vi "Word_Font_Wizard.vi"(3 "error in (no error)":errorcluster, 4 "font in":T1={"font name"="", "font size"=0.0, "bold"=0, "italic"=0, "underline"=0, "strike through"=0, "font color"=16777216} caption="font" {"font size" format="%0.2f"; "strike through" items=["Unchanged", "Yes", "No"]; "underline" items=["Unchanged", "Yes", "No"]; "italic" items=["Unchanged", "Yes", "No"]; "bold" items=["Unchanged", "Yes", "No"]}, 5 "Word._Application":refnum<k7>) -> (0 "error out":errorcluster, 1 "font out":T1={"font name"="", "font size"=0.0, "bold"=0, "italic"=0, "underline"=0, "strike through"=0, "font color"=16777216} caption="font" {"font size" format="%0.2f"; "strike through" items=["Unchanged", "Yes", "No"]; "underline" items=["Unchanged", "Yes", "No"]; "italic" items=["Unchanged", "Yes", "No"]; "bold" items=["Unchanged", "Yes", "No"]})   [LabVIEW 2020, in "NI_ReportGenerationToolkit.lvlib"]
uses:
  <vilib>/addons/_office/NI_ReportGenerationToolkit.lvlib
  <vilib>/addons/_office/_exclsub.llb/font.ctl
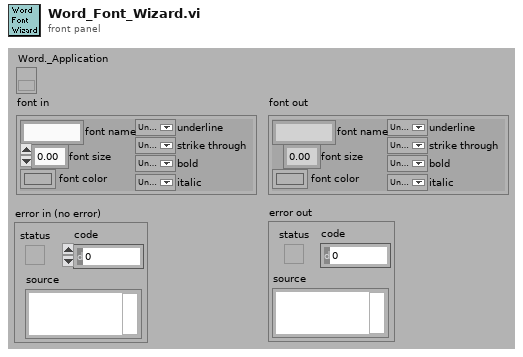
[diagram p1: front panel]
types:
  T1 = typedef "NI_ReportGenerationToolkit.lvlib/font.ctl" = cluster{"font name":string, "font size":dbl, "bold":u16, "italic":u16, "underline":u16, "strike through":u16, "font color":u32}
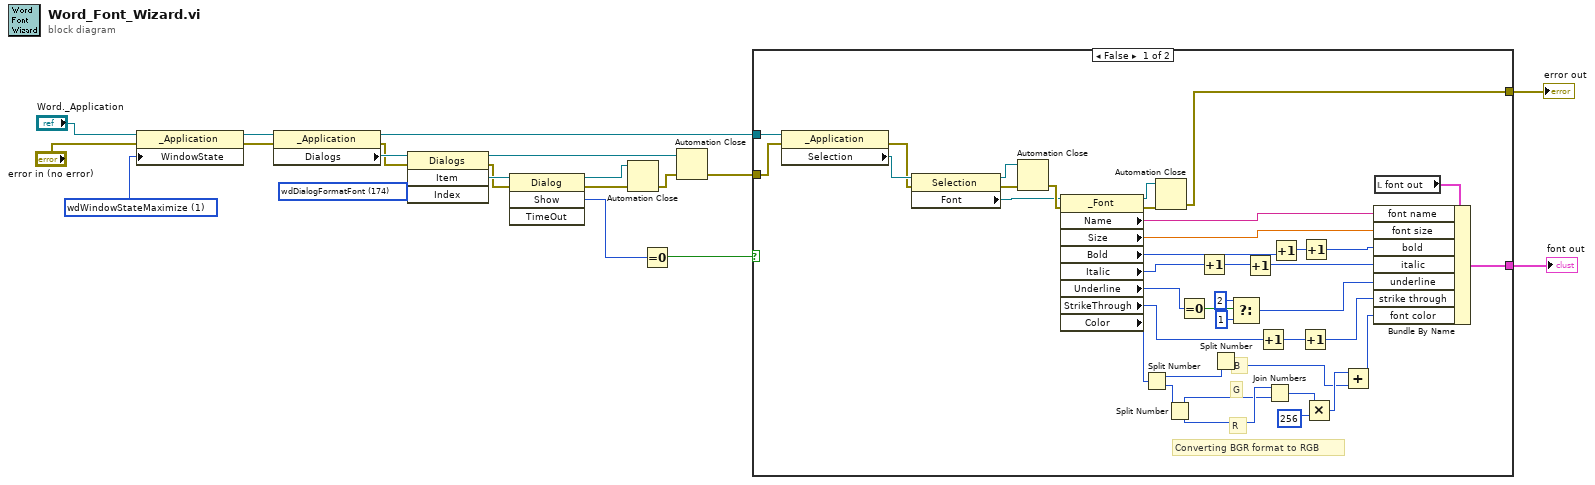
[diagram p0: block diagram]
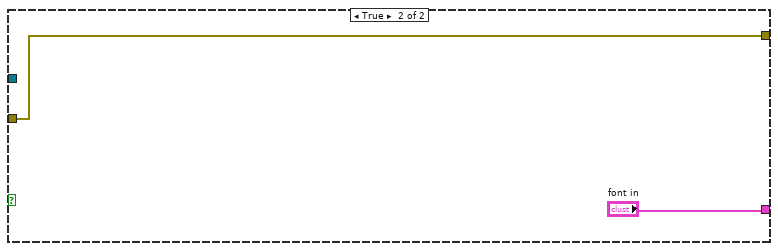
[diagram p2: hidden frame]
diagram:
  w6 = 1 items=["wdWindowStateNormal", "wdWindowStateMaximize", "wdWindowStateMinimize"] ("WindowState")
  w18 = 174 items=["wdDialogHelpAbout"=9, "wdDialogHelpWordPerfectHelp"=10, "wdDialogDocumentStatistics"=78, "wdDialogFileNew"=79, "wdDialogFileOpen"=80, "wdDialogMailMergeOpenDataSource"=81, "wdDialogMailMergeOpenHeaderSource"=82, "wdDialogFileSaveAs"=84, "wdDialogFileSummaryInfo"=86, "wdDialogToolsTemplates"=87, "wdDialogFilePrint"=88, "wdDialogFilePrintSetup"=97, "wdDialogFileFind"=99, "wdDialogFormatAddrFonts"=103, "wdDialogEditPasteSpecial"=111, "wdDialogEditFind"=112, "wdDialogEditReplace"=117, "wdDialogEditStyle"=120, "wdDialogEditLinks"=124, "wdDialogEditObject"=125, "wdDialogTableToText"=128, "wdDialogTextToTable"=127, "wdDialogTableInsertTable"=129, "wdDialogTableInsertCells"=130, "wdDialogTableInsertRow"=131, "wdDialogTableDeleteCells"=133, "wdDialogTableSplitCells"=137, "wdDialogTableRowHeight"=142, "wdDialogTableColumnWidth"=143, "wdDialogToolsCustomize"=152, "wdDialogInsertBreak"=159, "wdDialogInsertSymbol"=162, "wdDialogInsertPicture"=163, "wdDialogInsertFile"=164, "wdDialogInsertDateTime"=165, "wdDialogInsertField"=166, "wdDialogInsertMergeField"=167, "wdDialogInsertBookmark"=168, "wdDialogMarkIndexEntry"=169, "wdDialogInsertIndex"=170, "wdDialogInsertTableOfContents"=171, "wdDialogInsertObject"=172, "wdDialogToolsCreateEnvelope"=173, "wdDialogFormatFont"=174, "wdDialogFormatParagraph"=175, "wdDialogFormatSectionLayout"=176, "wdDialogFormatColumns"=177, "wdDialogFileDocumentLayout, wdDialogFilePageSetup"=178, "wdDialogFormatTabs"=179, "wdDialogFormatStyle"=180, "wdDialogFormatDefineStyleFont"=181, "wdDialogFormatDefineStylePara"=182, "wdDialogFormatDefineStyleTabs"=183, "wdDialogFormatDefineStyleFrame"=184, "wdDialogFormatDefineStyleBorders"=185, "wdDialogFormatDefineStyleLang"=186, "wdDialogFormatPicture"=187, "wdDialogToolsLanguage"=188, "wdDialogFormatBordersAndShading"=189, "wdDialogFormatFrame"=190, "wdDialogToolsThesaurus"=194, "wdDialogToolsHyphenation"=195, "wdDialogToolsBulletsNumbers"=196, "wdDialogToolsHighlightChanges, wdDialogToolsRevisions"=197, "wdDialogToolsCompareDocuments"=198, "wdDialogTableSort"=199, "wdDialogToolsOptionsGeneral"=203, "wdDialogToolsOptionsView"=204, "wdDialogToolsAdvancedSettings"=206, "wdDialogToolsOptionsPrint"=208, "wdDialogToolsOptionsSave"=209, "wdDialogToolsOptionsSpellingAndGrammar"=211, "wdDialogToolsOptionsUserInfo"=213, "wdDialogToolsMacroRecord"=214, "wdDialogToolsMacro"=215, "wdDialogWindowActivate"=220, "wdDialogFormatRetAddrFonts"=221, "wdDialogOrganizer"=222, "wdDialogToolsOptionsEdit"=224, "wdDialogToolsOptionsFileLocations"=225, "wdDialogToolsWordCount"=228, "wdDialogControlRun"=235, "wdDialogInsertPageNumbers"=294, "wdDialogFormatPageNumber"=298, "wdDialogCopyFile"=300, "wdDialogFormatChangeCase"=322, "wdDialogUpdateTOC"=331, "wdDialogInsertDatabase"=341, "wdDialogTableFormula"=348, "wdDialogFormFieldOptions"=353, "wdDialogInsertCaption"=357, "wdDialogInsertCaptionNumbering"=358, "wdDialogInsertAutoCaption"=359, "wdDialogFormFieldHelp"=361, "wdDialogInsertCrossReference"=367, "wdDialogInsertFootnote"=370, "wdDialogNoteOptions"=373, "wdDialogToolsAutoCorrect"=378, "wdDialogToolsOptionsTrackChanges"=386, "wdDialogConvertObject"=392, "wdDialogInsertAddCaption"=402, "wdDialogConnect"=420, "wdDialogToolsCustomizeKeyboard"=432, "wdDialogToolsCustomizeMenus"=433, "wdDialogToolsMergeDocuments"=435, "wdDialogMarkTableOfContentsEntry"=442, "wdDialogFileMacPageSetupGX"=444, "wdDialogFilePrintOneCopy"=445, "wdDialogEditFrame"=458, "wdDialogMarkCitation"=463, "wdDialogTableOfContentsOptions"=470, "wdDialogInsertTableOfAuthorities"=471, "wdDialogInsertTableOfFigures"=472, "wdDialogInsertIndexAndTables"=473, "wdDialogInsertFormField"=483, "wdDialogFormatDropCap"=488, "wdDialogToolsCreateLabels"=489, "wdDialogToolsProtectDocument"=503, "wdDialogFormatStyleGallery"=505, "wdDialogToolsAcceptRejectChanges"=506, "wdDialogHelpWordPerfectHelpOptions"=511, "wdDialogToolsUnprotectDocument"=521, "wdDialogToolsOptionsCompatibility"=525, "wdDialogTableOfCaptionsOptions"=551, "wdDialogTableAutoFormat"=563, "wdDialogMailMergeFindRecord"=569, "wdDialogReviewAfmtRevisions"=570, "wdDialogViewZoom"=577, "wdDialogToolsProtectSection"=578, "wdDialogFontSubstitution"=581, "wdDialogInsertSubdocument"=583, "wdDialogNewToolbar"=586, "wdDialogToolsEnvelopesAndLabels"=607, "wdDialogFormatCallout"=610, "wdDialogTableFormatCell"=612, "wdDialogToolsCustomizeMenuBar"=615, "wdDialogFileRoutingSlip"=624, "wdDialogEditTOACategory"=625, "wdDialogToolsManageFields"=631, "wdDialogDrawSnapToGrid"=633, "wdDialogDrawAlign"=634, "wdDialogMailMergeCreateDataSource"=642, "wdDialogMailMergeCreateHeaderSource"=643, "wdDialogMailMerge"=676, "wdDialogMailMergeCheck"=677, "wdDialogMailMergeHelper"=680, "wdDialogMailMergeQueryOptions"=681, "wdDialogFileMacPageSetup"=685, "wdDialogListCommands"=723, "wdDialogEditCreatePublisher"=732, "wdDialogEditSubscribeTo"=733, "wdDialogEditPublishOptions"=735, "wdDialogEditSubscribeOptions"=736, "wdDialogFileMacCustomPageSetupGX"=737, "wdDialogToolsOptionsTypography"=739, "wdDialogToolsAutoCorrectExceptions"=762, "wdDialogToolsOptionsAutoFormatAsYouType"=778, "wdDialogMailMergeUseAddressBook"=779, "wdDialogToolsHangulHanjaConversion"=784, "wdDialogToolsOptionsFuzzy"=790, "wdDialogEditGoToOld"=811, "wdDialogInsertNumber"=812, "wdDialogLetterWizard"=821, "wdDialogFormatBulletsAndNumbering"=824, "wdDialogToolsSpellingAndGrammar"=828, "wdDialogToolsCreateDirectory"=833, "wdDialogTableWrapping"=854, "wdDialogFormatTheme"=855, "wdDialogTableProperties"=861, "wdDialogEmailOptions"=863, "wdDialogCreateAutoText"=872, "wdDialogToolsAutoSummarize"=874, "wdDialogToolsGrammarSettings"=885, "wdDialogEditGoTo"=896, "wdDialogWebOptions"=898, "wdDialogInsertHyperlink"=925, "wdDialogToolsAutoManager"=915, "wdDialogFileVersions"=945, "wdDialogToolsOptionsAutoFormat"=959, "wdDialogFormatDrawingObject"=960, "wdDialogToolsOptions"=974, "wdDialogFitText"=983, "wdDialogEditAutoText"=985, "wdDialogPhoneticGuide"=986, "wdDialogToolsDictionary"=989, "wdDialogFileSaveVersion"=1007, "wdDialogToolsOptionsBidi"=1029, "wdDialogFrameSetProperties"=1074, "wdDialogTableTableOptions"=1080, "wdDialogTableCellOptions"=1081, "wdDialogIMESetDefault"=1094, "wdDialogTCSCTranslator"=1156, "wdDialogHorizontalInVertical"=1160, "wdDialogTwoLinesInOne"=1161, "wdDialogFormatEncloseCharacters"=1162, "wdDialogConsistencyChecker"=1121, "wdDialogToolsOptionsSmartTag"=1395, "wdDialogFormatStylesCustom"=1248, "wdDialogCSSLinks"=1261, "wdDialogInsertWebComponent"=1324, "wdDialogToolsOptionsEditCopyPaste"=1356, "wdDialogToolsOptionsSecurity"=1361, "wdDialogSearch"=1363, "wdDialogShowRepairs"=1381, "wdDialogMailMergeInsertAsk"=4047, "wdDialogMailMergeInsertFillIn"=4048, "wdDialogMailMergeInsertIf"=4049, "wdDialogMailMergeInsertNextIf"=4053, "wdDialogMailMergeInsertSet"=4054, "wdDialogMailMergeInsertSkipIf"=4055, "wdDialogMailMergeFieldMapping"=1304, "wdDialogMailMergeInsertAddressBlock"=1305, "wdDialogMailMergeInsertGreetingLine"=1306, "wdDialogMailMergeInsertFields"=1307, "wdDialogMailMergeRecipients"=1308, "wdDialogMailMergeFindRecipient"=1326, "wdDialogMailMergeSetDocumentType"=1339] ("Index")
  n1 = property class="_Application"(reference="Word._Application", error in="error in (no error)", "WindowState"=w6) -> (reference out=w2:refnum<k7>, error out=w1:errorcluster)
  n2 = property class="_Application"(reference=w2, error in=w1) -> (reference out=w12:refnum<k7>, error out=w19:errorcluster, "Dialogs"=w20:refnum<k7>)
  n3 = invoke class="Dialogs" method="Item"(reference=w20, error in=w19, "Index"=w18) -> (reference out=w13:refnum<k7>, error out=w16:errorcluster, "Item"=w17:refnum<k7>)  [unwired: 1 in, 1 out]
  n4 = invoke class="Dialog" method="Show"(reference=w17, error in=w16) -> (reference out=w14:refnum<k7>, error out=w15:errorcluster, "Show"=w11:i32)  [unwired: 2 in, 1 out]
  n5 = Automation Close(3:w15, 5:w14) -> (0:w10:errorcluster)
  n6 = Equal To 0?(x=w11) -> (x = 0?=w8:bool)
  n7 = Automation Close(3:w10, 5:w13) -> (0:w9:errorcluster)
  n8 = case shown="False" w8 {
    tunnel: [w21 w61] -> w5
    tunnel: w12 -> [w31 _]
    tunnel: w9 -> [w30 w61]
    tunnel: [w32 "font in"] -> w7
    frame False {
      # "Converting BGR format to RGB"
      # "R"
      # "G"
      # "B"
      n9 = property class="_Application"(reference=w31, error in=w30) -> (error out=w28:errorcluster, "Selection"=w29:refnum<k7>)  [unwired: 1 out]
      n10 = property class="Selection"(reference=w29, error in=w28) -> (reference out=w25:refnum<k7>, error out=w27:errorcluster, "Font"=w24:refnum<k7>)
      n11 = Automation Close(3:w27, 5:w25) -> (0:w26:errorcluster)
      n12 = property class="_Font"(reference=w24, error in=w26) -> (reference out=w22:refnum<k7>, error out=w23:errorcluster, "Name"=w58:string, "Size"=w57:sgl, "Bold"=w56:i32, "Italic"=w41:i32, "Underline"=w44:i32, "StrikeThrough"=w38:i32, "Color"=w47:i32)
      n13 = Split Number(x=w47) -> (hi(x)=w54:u16, lo(x)=w55:u16)
      n14 = Automation Close(3:w23, 5:w22) -> (0:w21:errorcluster)
      n15 = Split Number(x=w55) -> (hi(x)=w52:u8, lo(x)=w53:u8)
      n16 = Equal To 0?(x=w44) -> (x = 0?=w43:bool)
      n17 = Increment(x=w41) -> (x+1=w40:i32)
      n18 = Split Number(x=w54) -> (lo(x)=w48:u8)  [unwired: 1 out]
      n19 = Select(t=2, s=w43, f=1) -> (s? t:f=w35:i32)
      n20 = Increment(x=w40) -> (x+1=w39:i32)
      n21 = Increment(x=w38) -> (x+1=w37:i32)
      n22 = Join Numbers(hi=w53, lo=w52) -> ((hi.lo)=w51:u16)
      n23 = Increment(x=w56) -> (x+1=w34:i32)
      n24 = Increment(x=w37) -> (x+1=w36:i32)
      n25 = Increment(x=w34) -> (x+1=w33:i32)
      n26 = Multiply(x=w51, y=u32 256) -> (x*y=w49:u32)
      n27 = Add(x=w49, y=w48) -> (x+y=w46:u32)
      n28 = local read "font out"() -> (w59:T1)
      n29 = Bundle By Name(cluster=w59, "font name"=w58, "font size"=w57, "bold"=w33, "italic"=w39, "underline"=w35, "strike through"=w36, "font color"=w46) -> (w32:T1)
    }
    frame True {
    }
  }
  "error out" <- w5
  "font out" <- w7
